vi "configuration_exists.vi"(7 "configuration":refnum<vi>, 8 "error in (no error)":errorcluster, 9 "settings":string, 10 "configuration":string, 11 "class":path) -> (0 "error out":errorcluster)   [LabVIEW 2010, in "XComponentSpecification.xctl"]
uses:
  XComponentSpecification.xctl
  <vilib>/regexp/Match Regular Expression.xnode
  XUserDropdown/XUserDropdown/XUserDropdown.xctl
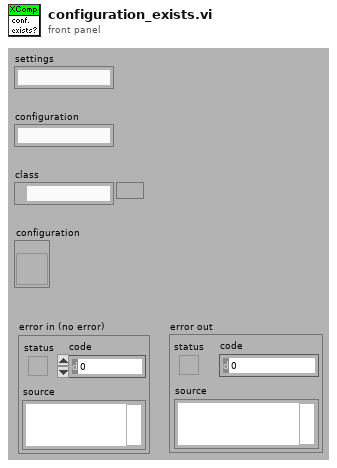
[diagram p1: front panel]
types:
  T1 = typedef "configuration_paths_cluster.ctl" = cluster{"base folder":path, "base folder for user":path, "component folder":path, "component file path":path, "main folder":path, "main file":path}
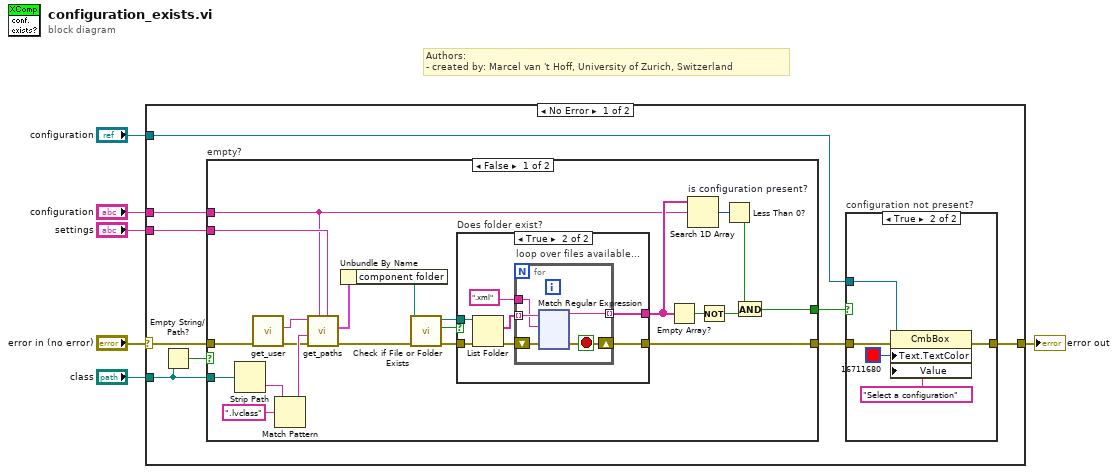
[diagram p0: block diagram]
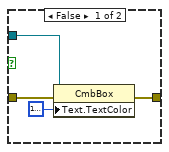
[diagram p2: hidden frame]
diagram:
  # "Authors: \n- created by: Marcel van 't Hoff, University of Zurich, Switzerland"
  n1 = case shown="No Error" "error in (no error)" {
    selector: "error in (no error)" -> [w9 w172]
    tunnel: "configuration" -> [w15 _]
    tunnel: "configuration" -> [w14 _]
    tunnel: "settings" -> [w13 _]
    tunnel: "class" -> [w10 _]
    tunnel: [w7 w172] -> w1
    frame No Error {
      n2 = Empty String/Path?(string/path=w10) -> (empty?=w11:bool)
      n3 = case "empty?" shown="False" w11 {
        tunnel: w10 -> [w44 _]
        tunnel: [w34 w171] -> w8
        tunnel: [w29 _] -> w12
        tunnel: w13 -> [w27 _]
        tunnel: w14 -> [w26 _]
        tunnel: w9 -> [w25 w171]
        frame False {
          n4 = Strip Path(path=w44) -> (name=w45:string)  [unwired: 1 out]
          n5 = call "get_user.vi"("error in (no error)"=w25) -> ("error out"=w38:errorcluster, "username out"=w42:string)  [unwired: 9 in]
          n6 = Match Pattern(string=w45, regular expression=".lvclass") -> (before substring=w43:string)  [unwired: 4 out]
          n7 = call "get_paths.vi"("settings file name (without ending)"=w27, "configuration file name (without ending)"=w26, "error in (no error)"=w38, "component name"=w43, "user"=w42) -> ("error out"=w39:errorcluster, "configuration paths"=w41:T1)  [unwired: 1 in, 4 out]
          n8 = Unbundle By Name(w41) -> ("component folder"=w40:path)
          n9 = call <vilib>:"Check if File or Folder Exists.vi"("error in (no error)"=w39, "path"=w40) -> ("error out"=w37:errorcluster, "file or folder exists?"=w35:bool, "dup path"=w36:path)  [unwired: 7 in]
          n10 = case "Does folder exist?" shown="True" w35 {
            tunnel: [w47 w49] -> w34
            tunnel: w36 -> [_ w51]
            tunnel: w37 -> [w47 w50]
            tunnel: [_ w48] -> w32
            frame False {
            }
            frame True {
              n11 = List Folder(path=w51, error in=w50) -> (filenames=w52:string[], error out=w53:errorcluster)  [unwired: 4 out]
              n12 = for "loop over files available..." {
                tunnel: w52 -> [w59] mode=indexing
                tunnel: [w58] -> w48 mode=indexing
                tunnel: ".xml" ("regular expression") -> [w56]
                shift-right: [w55] -> w49
                shift-left: w53 -> [w57]
                stop <- w55 stop-if-true
                n13 = xnode "Match Regular Expression"("input string"=w59, "regular expression"=w56, "error in"=w57) -> ("before match"=w58:string, "error out"=w55:errorcluster)  [unwired: 1 in, 5 out]
              }
            }
          }
          n14 = Empty Array?(array=w32) -> (empty?=w31:bool)
          n15 = Search 1D Array "is configuration present?"(1D array=w32, element=w26) -> (index of element=w33:i32)  [unwired: 1 in]
          n16 = Not(x=w31) -> (.not. x?=w28:bool)
          n17 = Less Than 0?(x=w33) -> (x < 0?=w30:bool)
          n18 = And(x=w30, y=w28) -> (x .and. y?=w29:bool)
        }
        frame True {
        }
      }
      n19 = case "configuration not present?" shown="True" w12 {
        tunnel: w15 -> [w18 w24]
        tunnel: w8 -> [w16 w21]
        tunnel: [w17 w20] -> w7
        frame False {
          n20 = property class="CmbBox"(reference=w18, error in=w16, "Text.TextColor"=u32 16777228 ("Color Box")) -> (error out=w17:errorcluster)  [unwired: 1 out]
        }
        frame True {
          n21 = property class="CmbBox"(reference=w24, error in=w21, "Text.TextColor"=u32 16711680, "Value"="Select a configuration") -> (error out=w20:errorcluster)  [unwired: 1 out]
        }
      }
    }
    frame Error {
    }
  }
  "error out" <- w1
